vi "Main.vi"(8 "error in":errorcluster, 11 "Debug Server in":refnum<class "Debug Server.lvclass">) -> (0 "error out":errorcluster, 3 "Debug Server out":refnum<class "Debug Server.lvclass">)   [LabVIEW 2017, in "Debug Server.lvclass"]
doc: "The <b>Queued Message Handler</b> of the Worker that owns this VI."
uses:
  Debug Server.lvclass
  C:/Program Files (x86)/National Instruments/LabVIEW 2017/vi.lib/addons/_Workers/Library/Classes/Worker/Worker.lvclass
  Debug Server.lvclass/Debug Server.ctl
  Initialization Data.ctl
  Settings/rqp_New Connection Log Message.ctl
  Application Manager/rqp_Display User Message.ctl
  Debug Server TCP Server and Client/Workers/DS TCP Server/rqp_Send Data to Debug Client.ctl
  Common VIs/DC_UID.ctl
  Message Log/rqp_Filter as Enque Worker.ctl
  Message Log/rqp_Filter as Deque Worker.ctl
  Application Manager/rqp_Open Running VI.ctl
  Application Manager/rqp_Go to MHL Case.ctl
  <vilib>/Utility/error.llb/Error Cluster From Error Code.vi
  <vilib>/ErrorRing/Error Ring.xnode
  Debug Server TCP Server and Client/Workers/DS TCP Server/DS TCP Server.lvclass
  Application Manager/Application Manager.lvclass
  Settings/Settings.lvclass
  Message Log/Message Log.lvclass
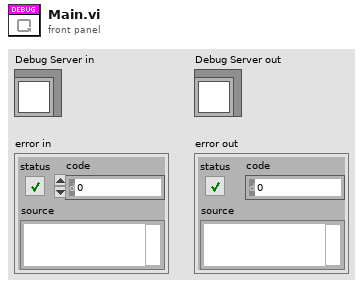
[diagram p1: front panel]
types:
  T1 = typedef "Debug Server.lvclass/Initialization Data.ctl" = cluster{"Placeholder - Can be deleted":string}
  T2 = typedef "Application Manager.lvclass/rqp_Display User Message.ctl" = cluster{"Message":string, "BG Color":u32}
  T3 = typedef "Settings.lvclass/rqp_New Connection Log Message.ctl" = cluster{"Message":string}
  T4 = typedef "DS TCP Server.lvlib/DS TCP Server.lvclass/rqp_Send Data to Debug Client.ctl" = cluster{"DC_UID":T5, "String to send":string}
  T5 = typedef "DC_UID.ctl" = string
  T6 = typedef "Message Log.lvclass/rqp_Filter as Enque Worker.ctl" = cluster{"Worker ID":string}
  T7 = typedef "Message Log.lvclass/rqp_Filter as Deque Worker.ctl" = cluster{"Worker ID":string}
  T8 = typedef "Application Manager.lvclass/rqp_Open Running VI.ctl" = cluster{"DC_UID":T5, "Worker ID":string}
  T9 = typedef "Application Manager.lvclass/rqp_Go to MHL Case.ctl" = cluster{"DC_UID":T5, "Worker ID":string, "Case Name":string}
  T10 = typedef "Application Manager.lvclass/rsp_Start Shutdown.ctl" = cluster{"Monitor":u16}
  T11 = typedef "Debug Server.lvclass/Dynamic Message Log Data.ctl" = cluster{"Message Log":refnum<class "Message Log.lvclass">, "DC_UID":T5, "Message Log ID":T12}
  T12 = typedef "Message Log ID.ctl" = cluster{"Head Worker ID":string, "IP Address":string}
  T13 = typedef "Application Manager.lvclass/rsp_Show Worker Front Panel.ctl" = cluster{"DC_UID":T5, "VI Path":path, "VI Ref":refnum<vi>}
  T14 = typedef "Application Manager.lvclass/rsp_Show Worker Block Diagram.ctl" = cluster{"DC_UID":T5, "VI Path":path, "VI Ref":refnum<vi>}
  T15 = typedef "Application Manager.lvclass/rsp_Send Start Exiting Request.ctl" = cluster{"DC_UID":T5, "Worker ID":string}
  T16 = typedef "Application Manager.lvclass/rsp_Filter as Enque Worker.ctl" = cluster{"Head Worker ID":string, "IP Address":string, "Worker ID":string}
  T17 = typedef "Application Manager.lvclass/rsp_Filter as Deque Worker.ctl" = cluster{"Head Worker ID":string, "IP Address":string, "Worker ID":string}
  T18 = typedef "Application Manager.lvclass/rsp_Go to MHL Case - Response.ctl" = cluster{"DC_UID":T5, "VI Path":path, "Case Name":string}
  T19 = typedef "Message Log.lvclass/rsp_Message Log Shutdown.ctl" = cluster{"Config Data":T20}
  T20 = typedef "Message Log.lvclass/Config Data.ctl" = cluster{"Max Num Rows":i32, "Visible Columns":bool[], "Splitter Position":i32, "Column Widths":u32[], "WinBounds":T21, "FP.State":enum32{"Invalid", "Standard", "Closed", "Hidden", "Minimized", "Maximized"}, "Monitor":u16, "Logging":bool, "LogBaseFolder":path}
  T21 = typedef "LVRectTypeDef.ctl" = cluster{"Left":i16, "Top":i16, "Right":i16, "Bottom":i16}
  T22 = enum32{"Invalid", "Standard", "Closed", "Hidden", "Minimized", "Maximized"}
  T23 = typedef "Message Log.lvclass/rsp_Open Running VI.ctl" = cluster{"Message Log ID":T12, "Worker ID":string}
  T24 = typedef "Message Log.lvclass/rsp_Go to MHL Case.ctl" = cluster{"Message Log ID":T12, "Worker ID":string, "Case Name":string}
  T25 = typedef "DS TCP Server.lvlib/DS TCP Server.lvclass/rsp_Server Port Open.ctl" = cluster{"Port":u16}
  T26 = typedef "DS TCP Server.lvlib/DS TCP Server.lvclass/rsp_Incompatible DC Connection.ctl" = cluster{"DC Version":string, "IP Address":string}
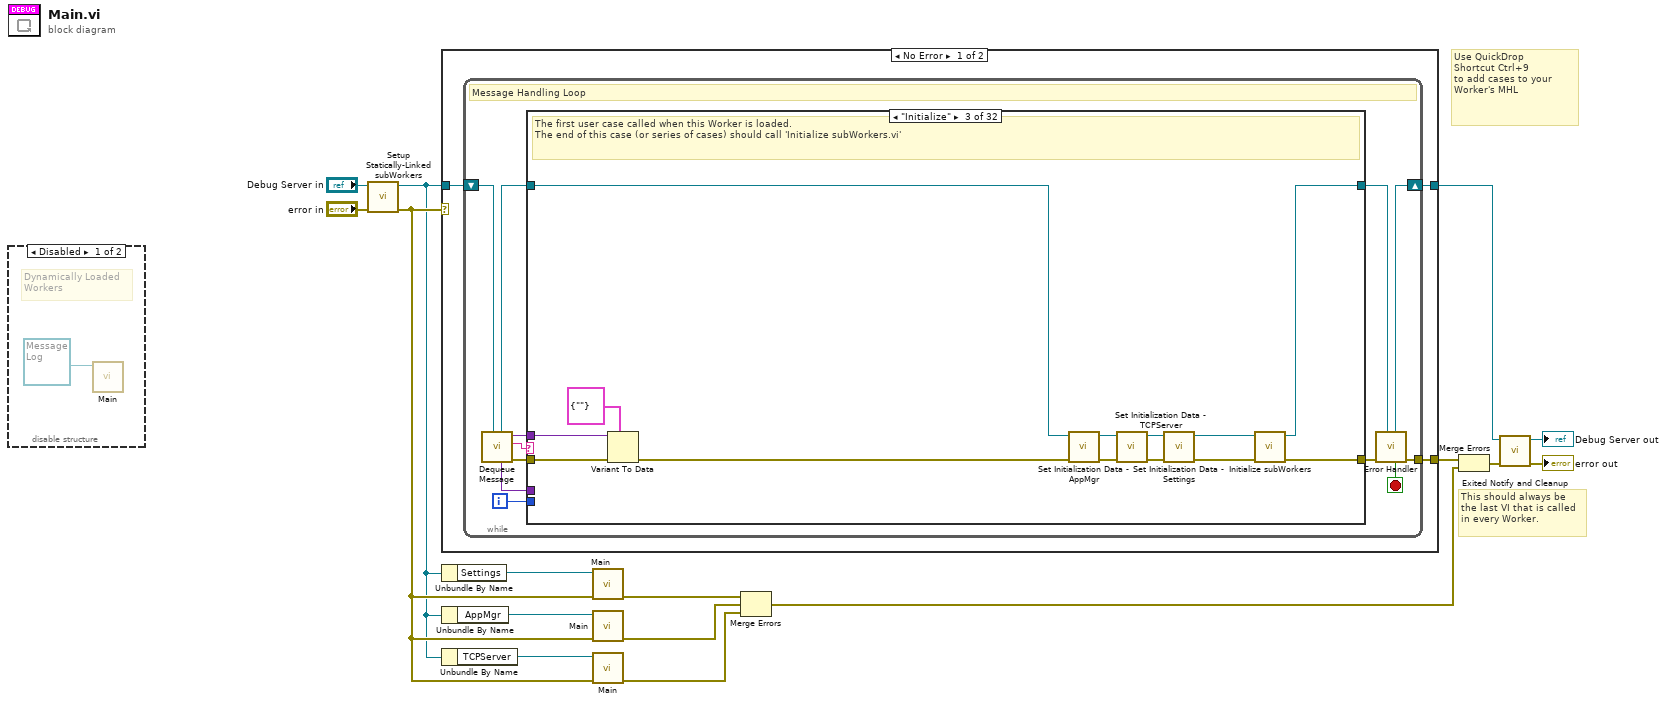
[diagram p0: block diagram]
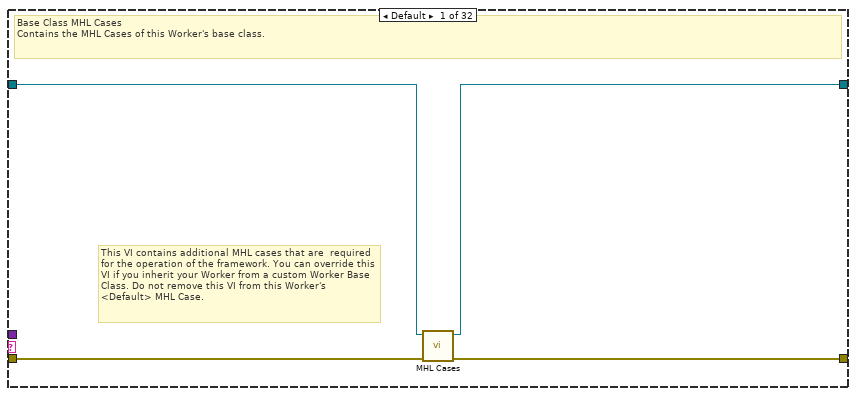
[diagram p3: hidden frame]
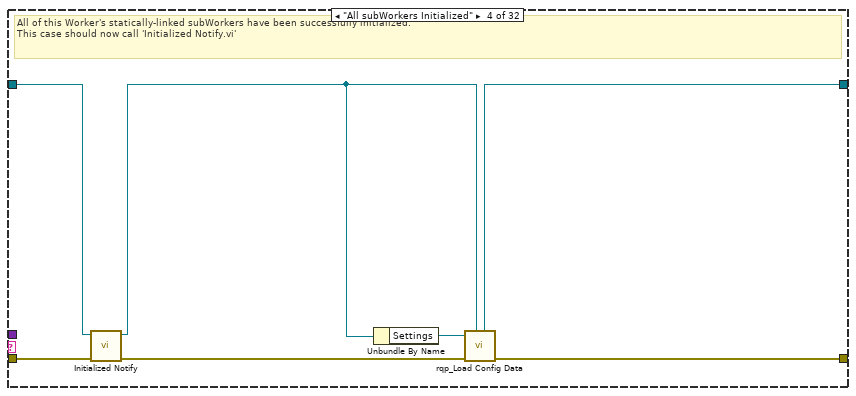
[diagram p5: hidden frame]
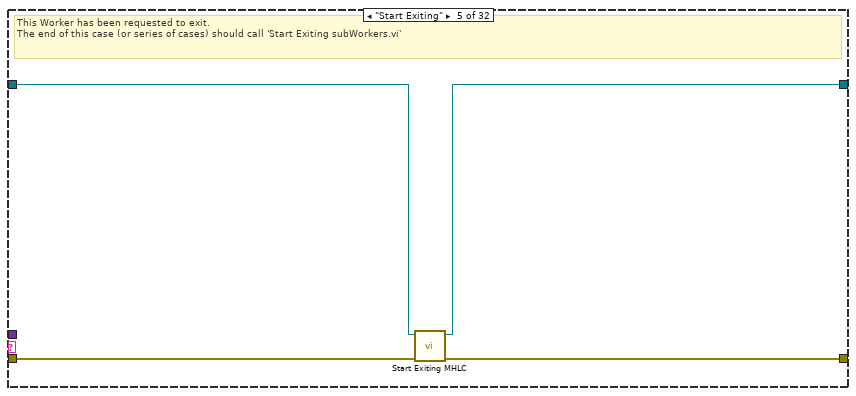
[diagram p6: hidden frame]
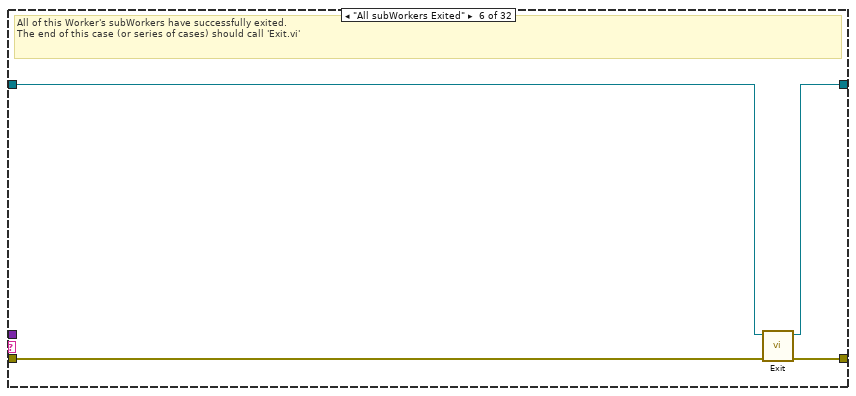
[diagram p7: hidden frame]
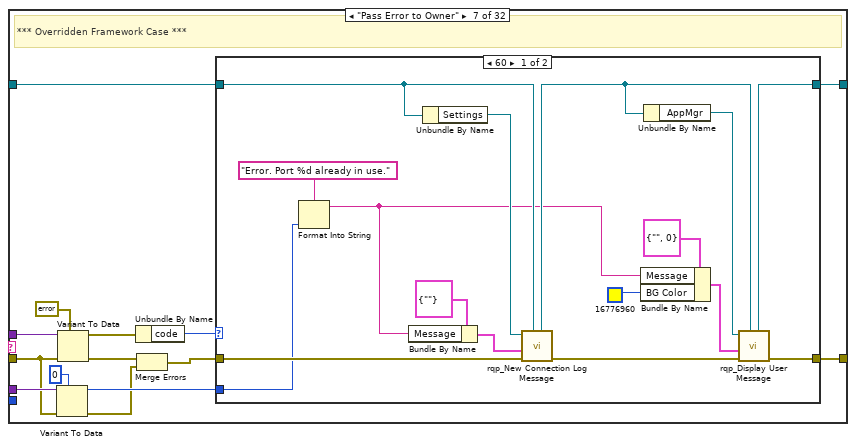
[diagram p8: hidden frame]
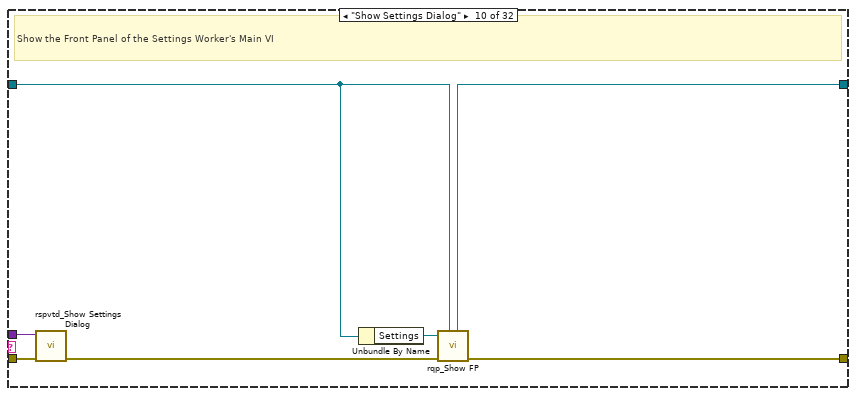
[diagram p12: hidden frame]
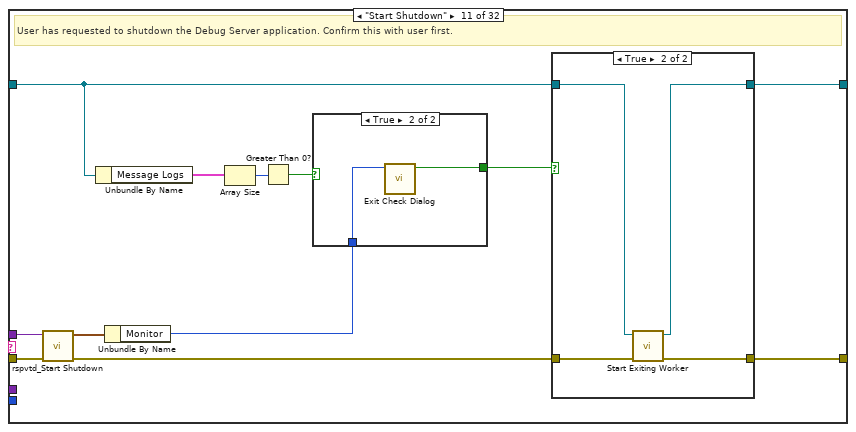
[diagram p13: hidden frame]
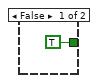
[diagram p15: hidden frame]
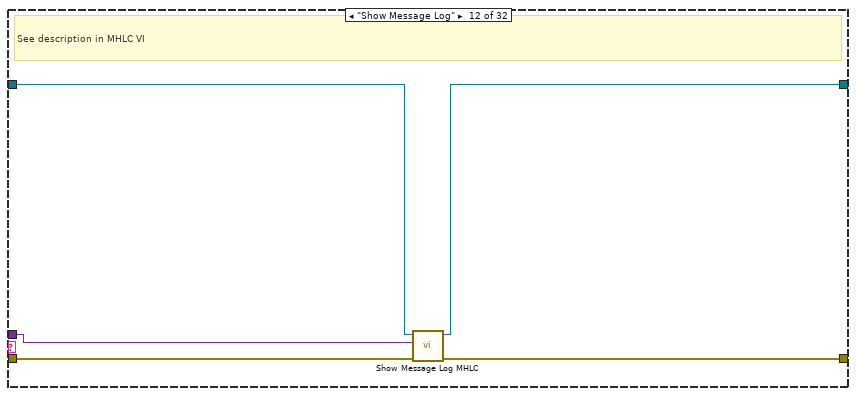
[diagram p16: hidden frame]
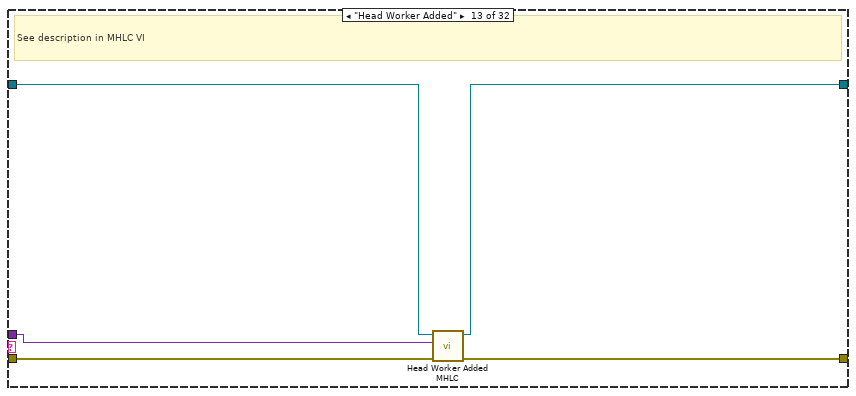
[diagram p17: hidden frame]
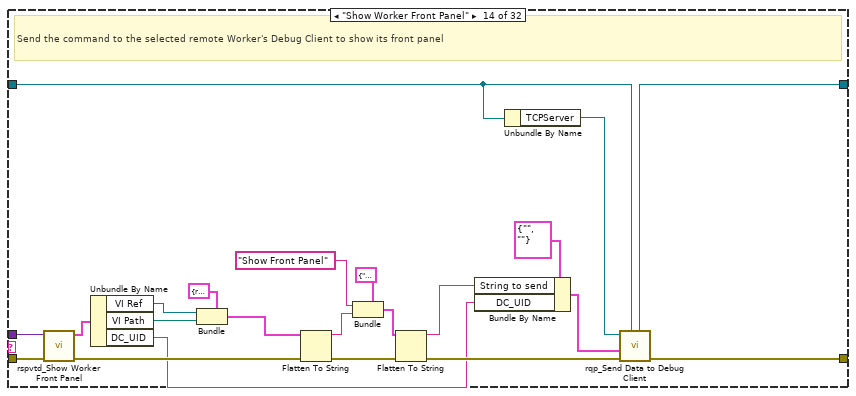
[diagram p18: hidden frame]
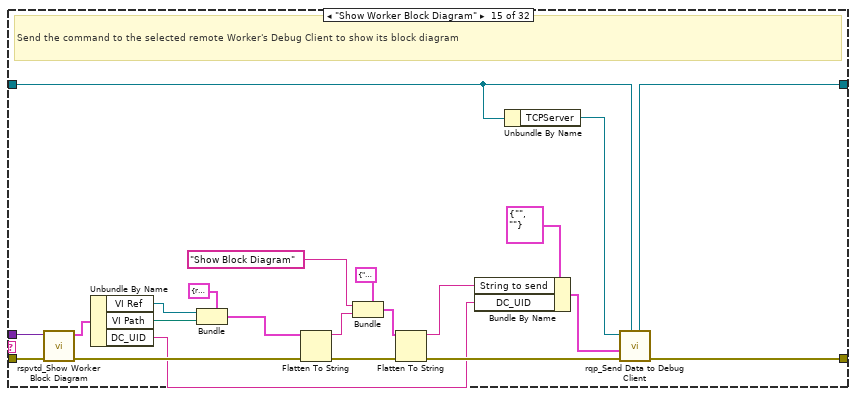
[diagram p19: hidden frame]
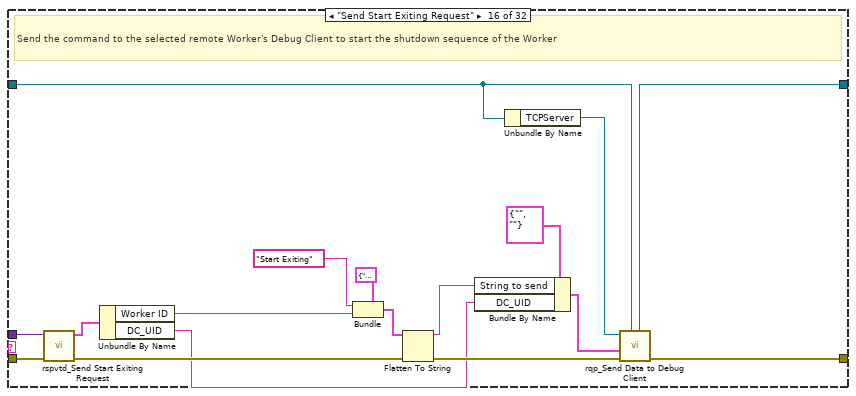
[diagram p20: hidden frame]
diagram:
  # "Use QuickDrop\nShortcut Ctrl+9\nto add cases to your\nWorker's MHL"
  # "This should always be the last VI that is called in every Worker."
  n1 = disable-structure shown="Disabled" {
    frame Disabled {
      # "Dynamically Loaded\nWorkers"
      n2 = call-dynamic "Main.vi"("Message Log in"=refnum<class "Message Log.lvclass"> refnum ("Message Log")) -> ()  [unwired: 9 in, 2 out]
    }
    frame Enabled {
    }
  }
  n3 = call "Setup Statically-Linked subWorkers.vi"("error in"="error in", "Debug Server in"="Debug Server in") -> ("error out"=w2:errorcluster, "Debug Server out"=w1:refnum<class "Debug Server.lvclass">)  [unwired: 8 in]
  n4 = case shown="No Error" w2 {
    tunnel: w1 -> [w20 w470]
    tunnel: [w18 w471] -> w14
    tunnel: [w19 w469] -> w15
    selector: w2 -> [_ w472]
    frame No Error {
      n5 = while {
        shift-right: [w30] -> w19
        shift-left: w20 -> [w32]
        tunnel: [w31] -> w18
        i -> [w22]
        stop <- w23 stop-if-true
        # "Message Handling Loop"
        n6 = call-dynamic "Dequeue Message.vi"("Worker"=w32) -> ("error out"=w29:errorcluster, "Case out"=w24:string, "Data out"=w25:variant, "Auxiliary out"=w21:variant, "Worker out"=w27:refnum<class "Debug Server.lvclass">)  [unwired: 6 in]
        n7 = case "Worker MHL Case Structure (DO NOT CHANGE LABEL NAME)" shown="\"Initialize\"" w24 {
          tunnel: w29 -> [w36 w37 w49 w57 w62 w66 w71 w100 w102 w109 w121 w135 w140 w162 w184 w201 w216 w259 w309 w311 w315 w322 w324 w329 w341 w354 w394 w428 w430 w449 w454 w468]
          tunnel: [w35 w37 w51 w55 w59 w65 w78 w100 w102 w106 w118 w134 w136 w159 w181 w198 w207 w250 w306 w311 w313 w319 w324 w327 w339 w347 w387 w427 w430 w439 w452 w458] -> w28
          tunnel: w27 -> [w34 w38 w41 w58 w61 w64 w74 w99 w101 w103 w115 w133 w138 w158 w180 w197 w209 w252 w305 w310 w314 w318 w323 w325 w340 w350 w390 w425 w429 w445 w450 w461]
          tunnel: [w33 w38 w50 w54 w60 w63 w73 w99 w101 w105 w117 w132 w137 w160 w182 w199 w210 w253 w307 w310 w312 w317 w323 w326 w337 w349 w389 w426 w429 w438 w451 w460] -> w26
          tunnel: w25 -> [_ _ w48 _ _ _ w79 _ _ w107 w119 w131 w139 w161 w183 w200 w215 w258 w308 _ w316 w320 _ w328 w338 w353 w393 w422 _ w447 w453 w467]
          tunnel: w22 -> [_ _ _ _ _ _ _ _ _ _ _ _ _ _ _ _ _ _ _ _ _ _ _ _ _ _ _ _ _ _ _ _]
          tunnel: w21 -> [_ _ _ _ _ _ w72 _ _ _ _ _ _ _ _ _ _ _ _ _ _ _ _ _ _ _ _ _ _ _ _ _]
          frame Default {
            # "This VI contains additional MHL cases that are  required for the operation of the framework. You can override this VI if you inherit your Worker from a custom Worker Base Class. Do not remove this VI from this Worker's <Default> MHL Case."
            # "Base Class MHL Cases\nContains the MHL Cases of this Worker's base class."
            n8 = call-dynamic "MHL Cases.vi"("error in"=w36, "Worker in"=w34) -> ("error out"=w35:errorcluster, "Worker out"=w33:refnum<class "Debug Server.lvclass">)  [unwired: 8 in]
          }
          frame "------------ FRAMEWORK CASES -----------" {
            # "Start of Workers Framework Cases"
          }
          frame "Initialize" {
            # "The first user case called when this Worker is loaded.\nThe end of this case (or series of cases) should call 'Initialize subWorkers.vi'"
            n9 = Variant To Data(error in=w49, type=T1 {"Placeholder - Can be deleted"=""} ("Initialization Data"), Variant=w48) -> (error out=w47:errorcluster)  [unwired: 1 out]
            n10 = call "Set Initialization Data - AppMgr.vi"("error in"=w47, "Debug Server in"=w41) -> ("error out"=w42:errorcluster, "Debug Server out"=w40:refnum<class "Debug Server.lvclass">)  [unwired: 8 in]
            n11 = call "Set Initialization Data - TCPServer.vi"("error in"=w42, "Debug Server in"=w40) -> ("error out"=w46:errorcluster, "Debug Server out"=w44:refnum<class "Debug Server.lvclass">)  [unwired: 8 in]
            n12 = call "Set Initialization Data - Settings.vi"("error in"=w46, "Debug Server in"=w44) -> ("error out"=w45:errorcluster, "Debug Server out"=w43:refnum<class "Debug Server.lvclass">)  [unwired: 8 in]
            n13 = call-dynamic "Initialize subWorkers.vi"("error in"=w45, "Worker"=w43) -> ("error out"=w51:errorcluster, "dup Worker out"=w50:refnum<class "Debug Server.lvclass">)  [unwired: 8 in]
          }
          frame "All subWorkers Initialized" {
            # "All of this Worker's statically-linked subWorkers have been successfully initialized.\nThis case should now call 'Initialized Notify.vi'"
            n14 = call-dynamic "Initialized Notify.vi"("error in"=w57, "Worker"=w58) -> ("error out"=w56:errorcluster, "dup Worker out"=w52:refnum<class "Debug Server.lvclass">)  [unwired: 8 in]
            n15 = Unbundle By Name(w52) -> ("Settings"=w53:refnum<class "Settings.lvclass">)
            n16 = call "rqp_Load Config Data.vi"("Caller in"=w52, "error in"=w56, "Settings in"=w53) -> ("error out"=w55:errorcluster, "dup Caller out"=w54:refnum<class "Debug Server.lvclass">)  [unwired: 6 in, 1 out]
          }
          frame "Start Exiting" {
            # "This Worker has been requested to exit. \nThe end of this case (or series of cases) should call 'Start Exiting subWorkers.vi'"
            n17 = call "Start Exiting MHLC.vi"("error in (no error)"=w62, "Debug Server in"=w61) -> ("error out"=w59:errorcluster, "Debug Server out"=w60:refnum<class "Debug Server.lvclass">)  [unwired: 8 in]
          }
          frame "All subWorkers Exited" {
            # "All of this Worker's subWorkers have successfully exited. \nThe end of this case (or series of cases) should call 'Exit.vi'"
            n18 = call-dynamic "Exit.vi"("error_in"=w66, "Worker"=w64) -> ("error out"=w65:errorcluster, "dup Worker out"=w63:refnum<class "Debug Server.lvclass">)  [unwired: 8 in]
          }
          frame "Pass Error to Owner" {
            # "*** Overridden Framework Case ***"
            n19 = Variant To Data(error in=w71, type=u16 0 ("Port"), Variant=w72) -> (data=w69:u16, error out=w67:errorcluster)
            n20 = Variant To Data(error in=w71, type=errorcluster {"status"=FALSE, "code"=0, "source"=""} ("error constant"), Variant=w79) -> (data=w76:errorcluster, error out=w77:errorcluster)
            n21 = Unbundle By Name(w76) -> ("code"=w75:i32)
            n22 = Merge Errors(w77, w67) -> (w68:errorcluster)
            n23 = case shown="60" w75 {
              tunnel: [w89 w98] -> w78
              tunnel: w68 -> [w96 w98]
              tunnel: w74 -> [w91 w97]
              tunnel: [w88 w97] -> w73
              tunnel: w69 -> [w92 _]
              frame 60 {
                n24 = Format Into String(format string="Error. Port %d already in use." ("Input String"), w92) -> (resulting string=w81:string)  [unwired: 2 in, 1 out]
                n25 = Bundle By Name(cluster=T3 {"Message"=""} ("Data in"), "Message"=w81) -> (w93:T3)
                n26 = Unbundle By Name(w91) -> ("Settings"=w90:refnum<class "Settings.lvclass">)
                n27 = call "rqp_New Connection Log Message.vi"("Caller in"=w91, "error in"=w96, "Data in"=w93, "Settings in"=w90) -> ("error out"=w95:errorcluster, "dup Caller out"=w87:refnum<class "Debug Server.lvclass">)  [unwired: 5 in, 1 out]
                n28 = Bundle By Name(cluster=T2 {"Message"="", "BG Color"=0} ("Data in"), "Message"=w81, "BG Color"=u32 16776960) -> (w84:T2)
                n29 = Unbundle By Name(w87) -> ("AppMgr"=w86:refnum<class "Application Manager.lvclass">)
                n30 = call "rqp_Display User Message.vi"("Caller in"=w87, "error in"=w95, "Data in"=w84, "Application Manager in"=w86) -> ("error out"=w89:errorcluster, "dup Caller out"=w88:refnum<class "Debug Server.lvclass">)  [unwired: 5 in, 1 out]
              }
              frame Default {
              }
            }
          }
          frame "------------- RESPONSE CASES --------------" {
            # "Start of Workers Response Cases"
          }
          frame " ---~~~~~~ Application Manager ~~~~~~ " {
            # "Start of registered Worker's Response Messages"
          }
          frame "Show Settings Dialog" {
            # "Show the Front Panel of the Settings Worker's Main VI"
            n31 = call "rspvtd_Show Settings Dialog.vi"("error in"=w109, "Data in"=w107) -> ("error out"=w108:errorcluster)  [unwired: 8 in, 1 out]
            n32 = Unbundle By Name(w103) -> ("Settings"=w104:refnum<class "Settings.lvclass">)
            n33 = call "rqp_Show FP.vi"("Caller in"=w103, "error in"=w108, "Settings in"=w104) -> ("error out"=w106:errorcluster, "dup Caller out"=w105:refnum<class "Debug Server.lvclass">)  [unwired: 6 in, 1 out]
          }
          frame "Start Shutdown" {
            # "User has requested to shutdown the Debug Server application. Confirm this with user first."
            n34 = call "rspvtd_Start Shutdown.vi"("error in"=w121, "Data in"=w119) -> ("error out"=w120:errorcluster, "Data out"=w116:T10)  [unwired: 8 in]
            n35 = Unbundle By Name(w115) -> ("Message Logs"=w114:T11[])
            n36 = Unbundle By Name(w116) -> ("Monitor"=w111:u16)
            n37 = Array Size(array=w114) -> (size(s)=w113:i32)
            n38 = Greater Than 0?(x=w113) -> (x > 0?=w112:bool)
            n39 = case shown="True" w112 {
              tunnel: w111 -> [_ w130]
              tunnel: [TRUE ("Exit?") w129] -> w110
              frame False {
              }
              frame True {
                n40 = call "Exit Check Dialog.vi"("Monitor"=w130) -> ("Exit?"=w129:bool)  [unwired: 10 in]
              }
            }
            n41 = case shown="True" w110 {
              tunnel: w120 -> [w122 w127]
              tunnel: [w122 w126] -> w118
              tunnel: [w123 w125] -> w117
              tunnel: w115 -> [w123 w124]
              frame False {
              }
              frame True {
                n42 = call-dynamic "Start Exiting Worker.vi"("error in"=w127, "Worker"=w124) -> ("error out"=w126:errorcluster, "dup Worker out"=w125:refnum<class "Debug Server.lvclass">)  [unwired: 8 in]
              }
            }
          }
          frame "Show Message Log" {
            # "See description in MHLC VI"
            n43 = call "Show Message Log MHLC.vi"("error in (no error)"=w135, "Data in"=w131, "Debug Server in"=w133) -> ("error out"=w134:errorcluster, "Debug Server out"=w132:refnum<class "Debug Server.lvclass">)  [unwired: 7 in]
          }
          frame "Head Worker Added" {
            # "See description in MHLC VI"
            n44 = call "Head Worker Added MHLC.vi"("error in (no error)"=w140, "Data in"=w139, "Debug Server in"=w138) -> ("error out"=w136:errorcluster, "Debug Server out"=w137:refnum<class "Debug Server.lvclass">)  [unwired: 7 in]
          }
          frame "Show Worker Front Panel" {
            # "Send the command to the selected remote Worker's Debug Client to show its front panel"
            n45 = call "rspvtd_Show Worker Front Panel.vi"("error in"=w162, "Data in"=w161) -> ("error out"=w144:errorcluster, "Data out"=w154:T13)  [unwired: 8 in]
            n46 = Unbundle By Name(w154) -> ("VI Ref"=w147:refnum<vi>, "VI Path"=w146:path, "DC_UID"=w141:T5)
            n47 = Bundle(cluster=cluster{"VI Ref":refnum<vi>, "VI Path":path} {"VI Ref"=refnum, "VI Path"=path ""}, "VI Ref"=w147, "VI Path"=w146) -> (w152:cluster{"VI Ref":refnum<vi>, "VI Path":path})
            n48 = Flatten To String(anything=w152, error in (no error)=w144) -> (data string=w153:string, error out=w148:errorcluster)  [unwired: 2 in, 1 out]
            n49 = Bundle(cluster=cluster{string, string} {"", ""}, "Show Front Panel", w153) -> (w149:cluster{string, string})
            n50 = Flatten To String(anything=w149, error in (no error)=w148) -> (data string=w155:string, error out=w143:errorcluster)  [unwired: 2 in, 1 out]
            n51 = Bundle By Name(cluster=T4 {"DC_UID"="", "String to send"=""} ("Data in"), "String to send"=w155, "DC_UID"=w141) -> (w142:T4)
            n52 = Unbundle By Name(w158) -> ("TCPServer"=w157:refnum<class "DS TCP Server.lvclass">)
            n53 = call "rqp_Send Data to Debug Client.vi"("Caller in"=w158, "error in"=w143, "Data in"=w142, "DS TCP Server in"=w157) -> ("error out"=w159:errorcluster, "dup Caller out"=w160:refnum<class "Debug Server.lvclass">)  [unwired: 5 in, 1 out]
          }
          frame "Show Worker Block Diagram" {
            # "Send the command to the selected remote Worker's Debug Client to show its block diagram"
            n54 = call "rspvtd_Show Worker Block Diagram.vi"("error in"=w184, "Data in"=w183) -> ("error out"=w166:errorcluster, "Data out"=w176:T14)  [unwired: 8 in]
            n55 = Unbundle By Name(w176) -> ("VI Ref"=w169:refnum<vi>, "VI Path"=w168:path, "DC_UID"=w163:T5)
            n56 = Bundle(cluster=cluster{"VI Ref":refnum<vi>, "VI Path":path} {"VI Ref"=refnum, "VI Path"=path ""}, "VI Ref"=w169, "VI Path"=w168) -> (w174:cluster{"VI Ref":refnum<vi>, "VI Path":path})
            n57 = Flatten To String(anything=w174, error in (no error)=w166) -> (data string=w175:string, error out=w170:errorcluster)  [unwired: 2 in, 1 out]
            n58 = Bundle(cluster=cluster{string, string} {"", ""}, "Show Block Diagram", w175) -> (w171:cluster{string, string})
            n59 = Flatten To String(anything=w171, error in (no error)=w170) -> (data string=w177:string, error out=w165:errorcluster)  [unwired: 2 in, 1 out]
            n60 = Bundle By Name(cluster=T4 {"DC_UID"="", "String to send"=""} ("Data in"), "String to send"=w177, "DC_UID"=w163) -> (w164:T4)
            n61 = Unbundle By Name(w180) -> ("TCPServer"=w179:refnum<class "DS TCP Server.lvclass">)
            n62 = call "rqp_Send Data to Debug Client.vi"("Caller in"=w180, "error in"=w165, "Data in"=w164, "DS TCP Server in"=w179) -> ("error out"=w181:errorcluster, "dup Caller out"=w182:refnum<class "Debug Server.lvclass">)  [unwired: 5 in, 1 out]
          }
          frame "Send Start Exiting Request" {
            # "Send the command to the selected remote Worker's Debug Client to start the shutdown sequence of the Worker"
            n63 = call "rspvtd_Send Start Exiting Request.vi"("error in"=w201, "Data in"=w200) -> ("error out"=w189:errorcluster, "Data out"=w193:T15)  [unwired: 8 in]
            n64 = Unbundle By Name(w193) -> ("Worker ID"=w185:string, "DC_UID"=w186:T5)
            n65 = Bundle(cluster=cluster{string, string} {"", ""}, "Start Exiting", w185) -> (w191:cluster{string, string})
            n66 = Flatten To String(anything=w191, error in (no error)=w189) -> (data string=w194:string, error out=w188:errorcluster)  [unwired: 2 in, 1 out]
            n67 = Bundle By Name(cluster=T4 {"DC_UID"="", "String to send"=""} ("Data in"), "String to send"=w194, "DC_UID"=w186) -> (w187:T4)
            n68 = Unbundle By Name(w197) -> ("TCPServer"=w196:refnum<class "DS TCP Server.lvclass">)
            n69 = call "rqp_Send Data to Debug Client.vi"("Caller in"=w197, "error in"=w188, "Data in"=w187, "DS TCP Server in"=w196) -> ("error out"=w198:errorcluster, "dup Caller out"=w199:refnum<class "Debug Server.lvclass">)  [unwired: 5 in, 1 out]
          }
          frame "Filter as Enque Worker" {
            # "If Message Log exists for selected Worker, apply filter using Worker as Enqueue Worker"
            n70 = call "rspvtd_Filter as Enque Worker.vi"("error in"=w216, "Data in"=w215) -> ("error out"=w208:errorcluster, "Data out"=w214:T16)  [unwired: 8 in]
            n71 = Unbundle By Name(w214) -> ("Head Worker ID"=w213:string, "IP Address"=w212:string, "Worker ID"=w202:string)
            n72 = Unbundle By Name(w209) -> ("Message Logs"=w211:T11[])
            n73 = call "Create Message Log ID.vi"("IP Address"=w212, "Head Worker WID"=w213) -> ("Message Log ID"=w205:T12)  [unwired: 9 in]
            n74 = for {
              tunnel: w211 -> [w244] mode=indexing
              tunnel: w205 -> [w242]
              tunnel: [w241] -> w206
              tunnel: [w240] -> w203
              stop <- w241 stop-if-true
              n75 = Unbundle By Name(w244) -> ("Message Log"=w240:refnum<class "Message Log.lvclass">, "Message Log ID"=w243:T12)
              n76 = Equal?(x=w243, y=w242) -> (x = y?=w241:bool)
            }
            n77 = call "Message Log ID to String.vi"("Message Log ID"=w205) -> ("Message Log ID String"=w204:string)  [unwired: 10 in]
            n78 = case shown="True" w206 {
              tunnel: [w221 w237] -> w210
              tunnel: w209 -> [w221 w235]
              tunnel: w208 -> [w220 w239]
              tunnel: [w219 w238] -> w207
              tunnel: w204 -> [w217 _]
              tunnel: w203 -> [_ w232]
              tunnel: w202 -> [_ w229]
              frame False {
                n79 = xnode "Error Ring"("parameter 0"=w217) -> ("error out"=w218:errorcluster)
                n80 = Merge Errors(w220, w218) -> (w219:errorcluster)
              }
              frame True {
                n81 = Bundle By Name(cluster=T6 {"Worker ID"=""} ("Data"), "Worker ID"=w229) -> (w230:T6)
                n82 = call "rqp_Filter as Enque Worker.vi"("Caller in"=w235, "error in"=w239, "Data in"=w230, "Message Log in"=w232) -> ("error out"=w236:errorcluster, "dup Message Log out"=w233:refnum<class "Message Log.lvclass">, "dup Caller out"=w234:refnum<class "Debug Server.lvclass">)  [unwired: 5 in]
                n83 = call "rqp_Show Front Panel.vi"("Caller in"=w234, "error in"=w236, "Message Log in"=w233) -> ("error out"=w238:errorcluster, "dup Caller out"=w237:refnum<class "Debug Server.lvclass">)  [unwired: 6 in, 1 out]
              }
            }
          }
          frame "Filter as Deque Worker" {
            # "If Message Log exists for selected Worker, apply filter using Worker as Dequeue Worker"
            n84 = call "rspvtd_Filter as Deque Worker.vi"("error in"=w259, "Data in"=w258) -> ("error out"=w251:errorcluster, "Data out"=w257:T17)  [unwired: 8 in]
            n85 = Unbundle By Name(w257) -> ("Head Worker ID"=w256:string, "IP Address"=w255:string, "Worker ID"=w245:string)
            n86 = Unbundle By Name(w252) -> ("Message Logs"=w254:T11[])
            n87 = call "Create Message Log ID.vi"("IP Address"=w255, "Head Worker WID"=w256) -> ("Message Log ID"=w248:T12)  [unwired: 9 in]
            n88 = for {
              tunnel: w254 -> [w287] mode=indexing
              tunnel: w248 -> [w285]
              tunnel: [w284] -> w249
              tunnel: [w283] -> w246
              stop <- w284 stop-if-true
              n89 = Unbundle By Name(w287) -> ("Message Log"=w283:refnum<class "Message Log.lvclass">, "Message Log ID"=w286:T12)
              n90 = Equal?(x=w286, y=w285) -> (x = y?=w284:bool)
            }
            n91 = call "Message Log ID to String.vi"("Message Log ID"=w248) -> ("Message Log ID String"=w247:string)  [unwired: 10 in]
            n92 = case shown="True" w249 {
              tunnel: [w264 w280] -> w253
              tunnel: w252 -> [w264 w278]
              tunnel: w251 -> [w263 w282]
              tunnel: [w262 w281] -> w250
              tunnel: w247 -> [w260 _]
              tunnel: w246 -> [_ w275]
              tunnel: w245 -> [_ w272]
              frame False {
                n93 = xnode "Error Ring"("parameter 0"=w260) -> ("error out"=w261:errorcluster)
                n94 = Merge Errors(w263, w261) -> (w262:errorcluster)
              }
              frame True {
                n95 = Bundle By Name(cluster=T7 {"Worker ID"=""} ("Data"), "Worker ID"=w272) -> (w273:T7)
                n96 = call "rqp_Filter as Deque Worker.vi"("Caller in"=w278, "error in"=w282, "Data in"=w273, "Message Log in"=w275) -> ("error out"=w279:errorcluster, "dup Message Log out"=w276:refnum<class "Message Log.lvclass">, "dup Caller out"=w277:refnum<class "Debug Server.lvclass">)  [unwired: 5 in]
                n97 = call "rqp_Show Front Panel.vi"("Caller in"=w277, "error in"=w279, "Message Log in"=w276) -> ("error out"=w281:errorcluster, "dup Caller out"=w280:refnum<class "Debug Server.lvclass">)  [unwired: 6 in, 1 out]
              }
            }
          }
          frame "Go to MHL Case - App Manager" {
            # "Send the command to the selected remote Worker's Debug Client to view the selected Worker's MHL case on its Main VI."
            n98 = call "rspvtd_Go to MHL Case - Response.vi"("error in"=w309, "Data in"=w308) -> ("error out"=w295:errorcluster, "Data out"=w301:T18)  [unwired: 8 in]
            n99 = Unbundle By Name(w301) -> ("VI Path"=w288:path, "Case Name"=w290:string, "DC_UID"=w292:T5)
            n100 = Bundle(cluster=cluster{"VI Path":path, "Status":string} {"VI Path"=path "", "Status"=""}, "VI Path"=w288, "Status"=w290) -> (w289:cluster{"VI Path":path, "Status":string})
            n101 = Flatten To String(anything=w289, error in (no error)=w295) -> (data string=w300:string, error out=w297:errorcluster)  [unwired: 2 in, 1 out]
            n102 = Bundle(cluster=cluster{string, string} {"", ""}, "Go to Case", w300) -> (w298:cluster{string, string})
            n103 = Flatten To String(anything=w298, error in (no error)=w297) -> (data string=w302:string, error out=w294:errorcluster)  [unwired: 2 in, 1 out]
            n104 = Bundle By Name(cluster=T4 {"DC_UID"="", "String to send"=""} ("Data in"), "String to send"=w302, "DC_UID"=w292) -> (w293:T4)
            n105 = Unbundle By Name(w305) -> ("TCPServer"=w304:refnum<class "DS TCP Server.lvclass">)
            n106 = call "rqp_Send Data to Debug Client.vi"("Caller in"=w305, "error in"=w294, "Data in"=w293, "DS TCP Server in"=w304) -> ("error out"=w306:errorcluster, "dup Caller out"=w307:refnum<class "Debug Server.lvclass">)  [unwired: 5 in, 1 out]
          }
          frame " ---~~~~~~ Settings ~~~~~~~~~~ " {
            # "Start of registered Worker's Response Messages"
          }
          frame "Configuration Data" {
            # "See description in MHLC VI"
            n107 = call "Configuration Data MHLC.vi"("error in (no error)"=w315, "Data in"=w316, "Debug Server in"=w314) -> ("error out"=w313:errorcluster, "Debug Server out"=w312:refnum<class "Debug Server.lvclass">)  [unwired: 7 in]
          }
          frame "Shutdown Data Written to File" {
            # "Shutdown data has been successfully written to file.\nStart the official shutdown routine of the entire Debug Server application."
            n108 = call "rspvtd_Shutdown Data Written to File.vi"("error in"=w322, "Data in"=w320) -> ("error out"=w321:errorcluster)  [unwired: 8 in, 1 out]
            n109 = call-dynamic "Start Exiting subWorkers.vi"("error_in"=w321, "Worker"=w318) -> ("error out"=w319:errorcluster, "dup Worker out"=w317:refnum<class "Debug Server.lvclass">)  [unwired: 8 in]
          }
          frame " ---~~~~~~ Message Log ~~~~~~ " {
            # "Start of registered Worker's Response Messages"
          }
          frame "Message Log Exited" {
            # "See description in MHLC VI"
            n110 = call "Message Log Exited MHLC.vi"("error in (no error)"=w329, "Data in"=w328, "Debug Server in"=w325) -> ("error out"=w327:errorcluster, "Debug Server out"=w326:refnum<class "Debug Server.lvclass">)  [unwired: 7 in]
          }
          frame "Message Log Shutdown Data" {
            # "This case is used to update the data from the last closed Message Log, so that the next opened\nMessage Log will open with the same configuration"
            n111 = call "rspvtd_Message Log Shutdown Data.vi"("error in"=w341, "Data in"=w338) -> ("error out"=w339:errorcluster, "Data out"=w336:T19)  [unwired: 8 in]
            n112 = Unbundle By Name(w336) -> ("Config Data.Visible Columns"=w335:bool[], "Config Data.Splitter Position"=w334:i32, "Config Data.Column Widths"=w333:u32[], "Config Data.WinBounds"=w332:T21, "Config Data.FP.State"=w331:T22, "Config Data.Monitor"=w330:u16)
            n113 = Bundle By Name(cluster=w340, "Visible ML Columns"=w335, "Splitter Position"=w334, "Column Widths"=w333, "WinBounds"=w332, "FP.State"=w331, "Monitor"=w330) -> (w337:refnum<class "Debug Server.lvclass">)
          }
          frame "Open Running VI" {
            # "Send Request to Application Manager to open the selected Worker's (clone) Main VI's running block diagram"
            n114 = call "rspvtd_Open Running VI.vi"("error in"=w354, "Data in"=w353) -> ("error out"=w348:errorcluster, "Data out"=w352:T23)  [unwired: 8 in]
            n115 = Unbundle By Name(w352) -> ("Message Log ID"=w345:T12, "Worker ID"=w342:string)
            n116 = Unbundle By Name(w350) -> ("Message Logs"=w351:T11[])
            n117 = for {
              tunnel: w351 -> [w380] mode=indexing
              tunnel: w345 -> [w378]
              tunnel: [w377] -> w346
              tunnel: [w376] -> w343
              stop <- w377 stop-if-true
              n118 = Unbundle By Name(w380) -> ("DC_UID"=w376:T5, "Message Log ID"=w379:T12)
              n119 = Equal?(x=w379, y=w378) -> (x = y?=w377:bool)
            }
            n120 = call "Message Log ID to String.vi"("Message Log ID"=w345) -> ("Message Log ID String"=w344:string)  [unwired: 10 in]
            n121 = case shown="True" w346 {
              tunnel: w350 -> [w359 w372]
              tunnel: [w359 w373] -> w349
              tunnel: w348 -> [w358 w375]
              tunnel: [w357 w374] -> w347
              tunnel: w344 -> [w356 _]
              tunnel: w343 -> [_ w368]
              tunnel: w342 -> [_ w367]
              frame False {
                n122 = xnode "Error Ring"("parameter 0"=w356) -> ("error out"=w355:errorcluster)
                n123 = Merge Errors(w358, w355) -> (w357:errorcluster)
              }
              frame True {
                n124 = Bundle By Name(cluster=T8 {"DC_UID"="", "Worker ID"=""} ("Data in"), "DC_UID"=w368, "Worker ID"=w367) -> (w369:T8)
                n125 = Unbundle By Name(w372) -> ("AppMgr"=w371:refnum<class "Application Manager.lvclass">)
                n126 = call "rqp_Open Running VI.vi"("Caller in"=w372, "error in"=w375, "Data in"=w369, "Application Manager in"=w371) -> ("error out"=w374:errorcluster, "dup Caller out"=w373:refnum<class "Debug Server.lvclass">)  [unwired: 5 in, 1 out]
              }
            }
          }
          frame "Go to MHL Case" {
            # "Send Request to Application Manager to open the selected Worker's selected MHL Case on its Main VI"
            n127 = call "rspvtd_Go to MHL Case.vi"("error in"=w394, "Data in"=w393) -> ("error out"=w388:errorcluster, "Data out"=w392:T24)  [unwired: 8 in]
            n128 = Unbundle By Name(w392) -> ("Message Log ID"=w385:T12, "Worker ID"=w382:string, "Case Name"=w381:string)
            n129 = Unbundle By Name(w390) -> ("Message Logs"=w391:T11[])
            n130 = for {
              tunnel: w391 -> [w421] mode=indexing
              tunnel: w385 -> [w419]
              tunnel: [w418] -> w386
              tunnel: [w417] -> w383
              stop <- w418 stop-if-true
              n131 = Unbundle By Name(w421) -> ("DC_UID"=w417:T5, "Message Log ID"=w420:T12)
              n132 = Equal?(x=w420, y=w419) -> (x = y?=w418:bool)
            }
            n133 = call "Message Log ID to String.vi"("Message Log ID"=w385) -> ("Message Log ID String"=w384:string)  [unwired: 10 in]
            n134 = case shown="True" w386 {
              tunnel: w390 -> [w399 w413]
              tunnel: [w399 w414] -> w389
              tunnel: w388 -> [w398 w416]
              tunnel: [w397 w415] -> w387
              tunnel: w384 -> [w396 _]
              tunnel: w383 -> [_ w409]
              tunnel: w382 -> [_ w408]
              tunnel: w381 -> [_ w407]
              frame False {
                n135 = xnode "Error Ring"("parameter 0"=w396) -> ("error out"=w395:errorcluster)
                n136 = Merge Errors(w398, w395) -> (w397:errorcluster)
              }
              frame True {
                n137 = Bundle By Name(cluster=T9 {"DC_UID"="", "Worker ID"="", "Case Name"=""} ("Data in"), "DC_UID"=w409, "Worker ID"=w408, "Case Name"=w407) -> (w410:T9)
                n138 = Unbundle By Name(w413) -> ("AppMgr"=w412:refnum<class "Application Manager.lvclass">)
                n139 = call "rqp_Go to MHL Case.vi"("Caller in"=w413, "error in"=w416, "Data in"=w410, "Application Manager in"=w412) -> ("error out"=w415:errorcluster, "dup Caller out"=w414:refnum<class "Debug Server.lvclass">)  [unwired: 5 in, 1 out]
              }
            }
          }
          frame "Show Application Manager" {
            # "Open the front panel of the Application Manager"
            n140 = call "rspvtd_Show Application Manager.vi"("error in"=w428, "Data in"=w422) -> ("error out"=w423:errorcluster)  [unwired: 8 in, 1 out]
            n141 = Unbundle By Name(w425) -> ("AppMgr"=w424:refnum<class "Application Manager.lvclass">)
            n142 = call "rqp_Show Front Panel.vi"("Caller in"=w425, "error in"=w423, "Application Manager in"=w424) -> ("error out"=w427:errorcluster, "dup Caller out"=w426:refnum<class "Debug Server.lvclass">)  [unwired: 6 in, 1 out]
          }
          frame " ---~~~~~~ TCP Server ~~~~~~~~~~~ " {
            # "Start of registered Worker's Response Messages"
          }
          frame "Server Port Open" {
            # "TCP Server is listening on returned Port. Update this information to both Applicaiton Manager and Settings Workers."
            n143 = call "rspvtd_Server Port Open.vi"("error in"=w449, "Data in"=w447) -> ("error out"=w448:errorcluster, "Data out"=w443:T25)  [unwired: 8 in]
            n144 = Unbundle By Name(w443) -> ("Port"=w442:u16)
            n145 = Format Into String(format string="Server listening on port %d" ("Input String"), w442) -> (resulting string=w431:string)  [unwired: 2 in, 1 out]
            n146 = Bundle By Name(cluster=T3 {"Message"=""} ("Data in"), "Message"=w431) -> (w440:T3)
            n147 = Unbundle By Name(w445) -> ("Settings"=w444:refnum<class "Settings.lvclass">)
            n148 = call "rqp_New Connection Log Message.vi"("Caller in"=w445, "error in"=w448, "Data in"=w440, "Settings in"=w444) -> ("error out"=w446:errorcluster, "dup Caller out"=w435:refnum<class "Debug Server.lvclass">)  [unwired: 5 in, 1 out]
            n149 = Bundle By Name(cluster=T2 {"Message"="", "BG Color"=0} ("Data in"), "Message"=w431, "BG Color"=u32 16777216) -> (w433:T2)
            n150 = Unbundle By Name(w435) -> ("AppMgr"=w434:refnum<class "Application Manager.lvclass">)
            n151 = call "rqp_Display User Message.vi"("Caller in"=w435, "error in"=w446, "Data in"=w433, "Application Manager in"=w434) -> ("error out"=w439:errorcluster, "dup Caller out"=w438:refnum<class "Debug Server.lvclass">)  [unwired: 5 in, 1 out]
          }
          frame "Connection Notify" {
            # "See description in MHLC VI"
            n152 = call "Connection Notify MHLC.vi"("error in (no error)"=w454, "Data in"=w453, "Debug Server in"=w450) -> ("error out"=w452:errorcluster, "Debug Server out"=w451:refnum<class "Debug Server.lvclass">)  [unwired: 7 in]
          }
          frame "Incompatible DC Connection" {
            # "A connection to the Debug Server from a non-compatible Debug Client (wrong version) has been attempted. Send this message to Settings Worker."
            n153 = call "rspvtd_Incompatible DC Connection.vi"("error in"=w468, "Data in"=w467) -> ("error out"=w459:errorcluster, "Data out"=w457:T26)  [unwired: 8 in]
            n154 = Unbundle By Name(w457) -> ("DC Version"=w455:string, "IP Address"=w456:string)
            n155 = Format Into String(format string="An incompatible (Workers v%s) Debug Client attempted to connect to the Debug Server from %s." ("Input String"), w455, w456) -> (resulting string=w463:string)  [unwired: 2 in, 1 out]
            n156 = Bundle By Name(cluster=T3 {"Message"=""} ("Data in"), "Message"=w463) -> (w465:T3)
            n157 = Unbundle By Name(w461) -> ("Settings"=w462:refnum<class "Settings.lvclass">)
            n158 = call "rqp_New Connection Log Message.vi"("Caller in"=w461, "error in"=w459, "Data in"=w465, "Settings in"=w462) -> ("error out"=w458:errorcluster, "dup Caller out"=w460:refnum<class "Debug Server.lvclass">)  [unwired: 5 in, 1 out]
          }
        }
        n159 = call-dynamic "Error Handler.vi"("Worker"=w26, "error_in"=w28) -> ("error out"=w31:errorcluster, "Stop Loop"=w23:bool, "Worker out"=w30:refnum<class "Debug Server.lvclass">)  [unwired: 7 in]
      }
    }
    frame Error {
      n160 = call-dynamic "Error Handler.vi"("Worker"=w470, "error_in"=w472) -> ("error out"=w471:errorcluster, "Worker out"=w469:refnum<class "Debug Server.lvclass">)  [unwired: 7 in, 1 out]
    }
  }
  n161 = Unbundle By Name(w1) -> ("Settings"=w8:refnum<class "Settings.lvclass">)
  n162 = Unbundle By Name(w1) -> ("AppMgr"=w6:refnum<class "Application Manager.lvclass">)
  n163 = Unbundle By Name(w1) -> ("TCPServer"=w4:refnum<class "DS TCP Server.lvclass">)
  n164 = call-dynamic "Main.vi"("error in"=w2, "Settings in"=w8) -> ("error out"=w10:errorcluster)  [unwired: 8 in, 1 out]
  n165 = call-dynamic "Main.vi"("error in"=w2, "Application Manager in"=w6) -> ("error out"=w7:errorcluster)  [unwired: 8 in, 1 out]
  n166 = call-dynamic "Main.vi"("error in"=w2, "DS TCP Server in"=w4) -> ("error out"=w5:errorcluster)  [unwired: 8 in, 1 out]
  n167 = Merge Errors(w10, w7, w5) -> (w9:errorcluster)
  n168 = Merge Errors(w14, w9) -> (w16:errorcluster)
  n169 = call-dynamic "Exited Notify and Cleanup.vi"("error_in"=w16, "Worker"=w15) -> ("error out"=→"error out":errorcluster, "dup Worker out"=→"Debug Server out":refnum<class "Debug Server.lvclass">)  [unwired: 8 in]
